vi "FTW-Connector-LaunchActor.vi"(0 "FTW Actor Connector Type":refnum<class "FTW-ActorConnector.lvclass">, 5 "Actor VI Filepath":path, 7 "Configuration":T1, 11 "error in":errorcluster) -> (4 "FTW Actor Connector":refnum<class "FTW-ActorConnector.lvclass">, 15 "error out":errorcluster)   [LabVIEW 2012, in "FTW-Actor.lvlib" / "FTW-ActorConnector.lvclass"]
uses:
  FTW-ActorConnector.lvclass
  Utility/FTW-Actor-Configuration.ctl
  Core/src/JSON/FTW-JSON-RegexParse.vi
  Core/src/Regex/FTW-Regex.vi
  Core/src/JSON/FTW-JSON-RegexHeader.vi
  Core/src/Error/FTW-ERR-ThrowError.vi
  Core/src/Error/FTW-ERR-ThrowGenericError.vi
  Core/src/Container/FTW-Container-Construct.vi
  Core/src/Container/FTW-Container-Load-JSON.vi
  Core/src/Container/FTW-Container-Destroy.vi
  Core/src/JSON/FTW-JSON-Deserialize.xnode
  FTW-Actor.lvlib
  Core/src/Container/FTW-Container.lvclass
panel:
  # "Inputs"
  # "Outputs"
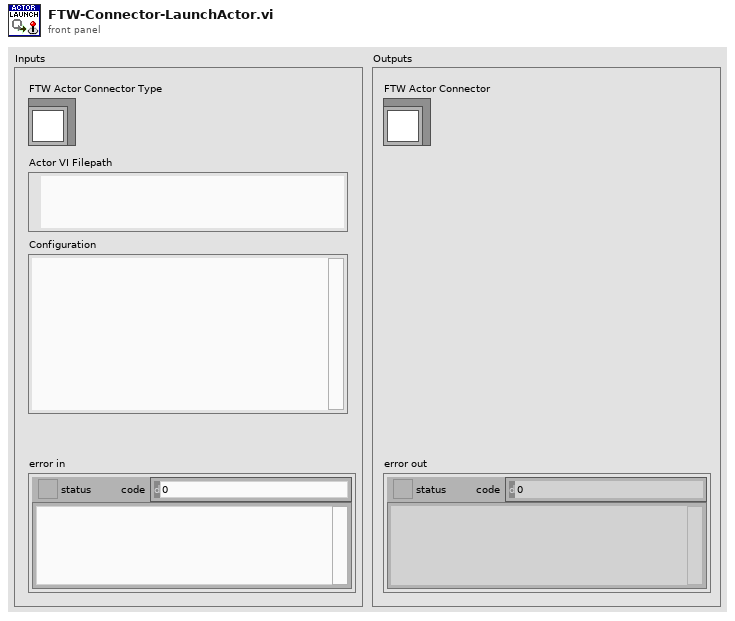
[diagram p1: front panel]
types:
  T1 = typedef "FTW-Actor.lvlib/FTW-Actor-Configuration.ctl" = string
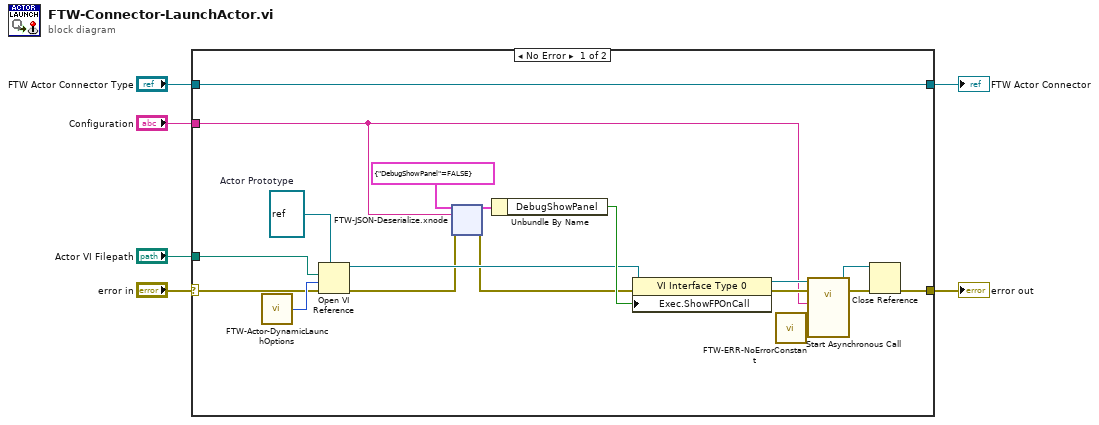
[diagram p0: block diagram]
diagram:
  n1 = case shown="No Error" "error in" {
    selector: "error in" -> [w20 w59]
    tunnel: [w22 w59] -> w6
    tunnel: "Configuration" -> [w9 _]
    tunnel: [w21 w58] -> w3
    tunnel: "FTW Actor Connector Type" -> [w21 w58]
    tunnel: "Actor VI Filepath" -> [w19 _]
    frame No Error {
      w24 = refnum<vi> refnum  # Actor Prototype
      n2 = call "FTW-Actor-DynamicLaunchOptions.vi"() -> ("Open VI Ref Options"=w23:i32)
      n3 = Open VI Reference(type specifier VI Refnum (for type only)=w24, vi path=w19, options=w23, error in (no error)=w20) -> (vi reference=w12:refnum<vi>, error out=w8:errorcluster)  [unwired: 2 in]
      n4 = xnode "FTW-JSON-Deserialize.xnode"("Data Type and Default Values"=cluster{"DebugShowPanel":bool} {"DebugShowPanel"=FALSE}, "JSON String"=w9, "error in"=w8) -> ("Populated Values"=w10:cluster{"DebugShowPanel":bool}, "error out"=w7:errorcluster)
      n5 = Unbundle By Name(w10) -> ("DebugShowPanel"=w13:bool)
      n6 = property class="VI Interface Type 0"(reference=w12, error in=w7, "Exec.ShowFPOnCall"=w13) -> (reference out=w15:refnum<vi>, error out=w14:errorcluster)
      n7 = call "FTW-ERR-NoErrorConstant.vi"() -> ("no error"=w18:errorcluster)
      n8 = call-by-ref "Start Asynchronous Call"(reference=w15, error in=w14, "Configuration"=w9, "ErrorIn"=w18) -> (reference out=w17:refnum<vi>, error out=w16:errorcluster)  [unwired: 13 in, 1 out]
      n9 = Close Reference(reference=w17, error in (no error)=w16) -> (error out=w22:errorcluster)
    }
    frame Error {
    }
  }
  "error out" <- w6
  "FTW Actor Connector" <- w3
